vi "Scale Rotated Recangle.vi"(0 "Scaled(%)":sgl, 1 "Type":enum16{"Image", "Text"}(ring), 2 "Automatic":bool, 5 "Original Rectangle":cluster{"width":dbl, "height":dbl}, 7 "Angle (rad)":dbl, 9 "Page or text zone size":cluster{"width":dbl, "height":dbl}, 11 "error in (no error)":errorcluster) -> (4 "Scale Factor (%)":dbl, 6 "Scale Factor":dbl, 8 "Scaled Rectangle":cluster{"width":dbl, "height":dbl}, 10 "Offset":cluster{"X":dbl, "Y":dbl}, 15 "error out":errorcluster)   [LabVIEW 2013]
doc: "Version 1.0\nDeveloped by Jean-Marc Simard\nCopyright © 2010, Exaprom Inc.\nAll rights reserved.\nLicense: BSD"
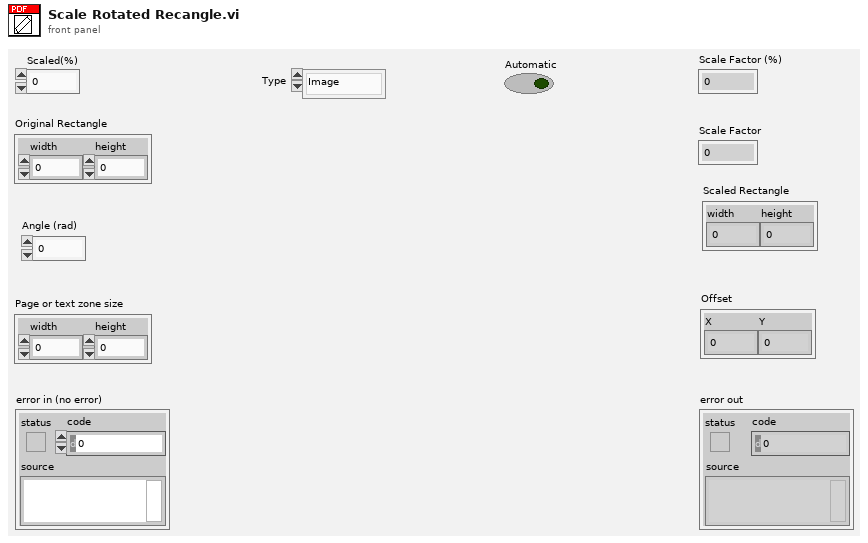
[diagram p1: front panel]
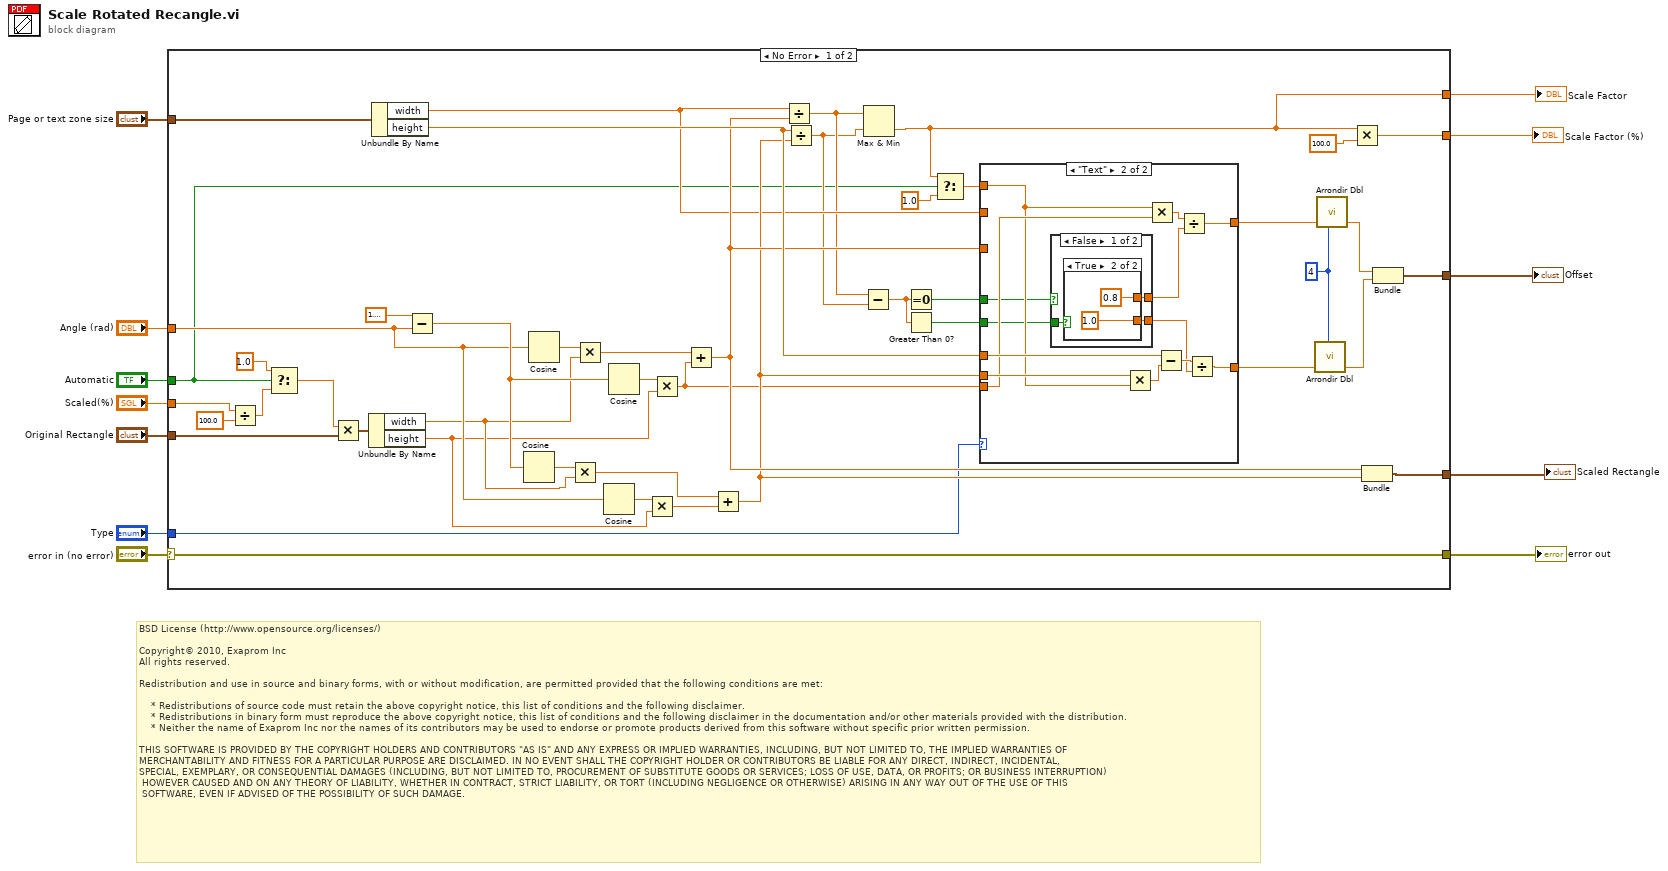
[diagram p0: block diagram]
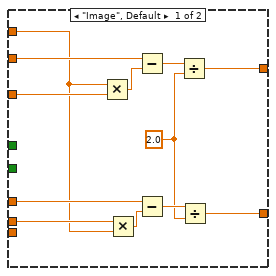
[diagram p2: hidden frame]
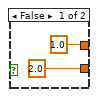
[diagram p3: hidden frame]
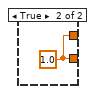
[diagram p4: hidden frame]
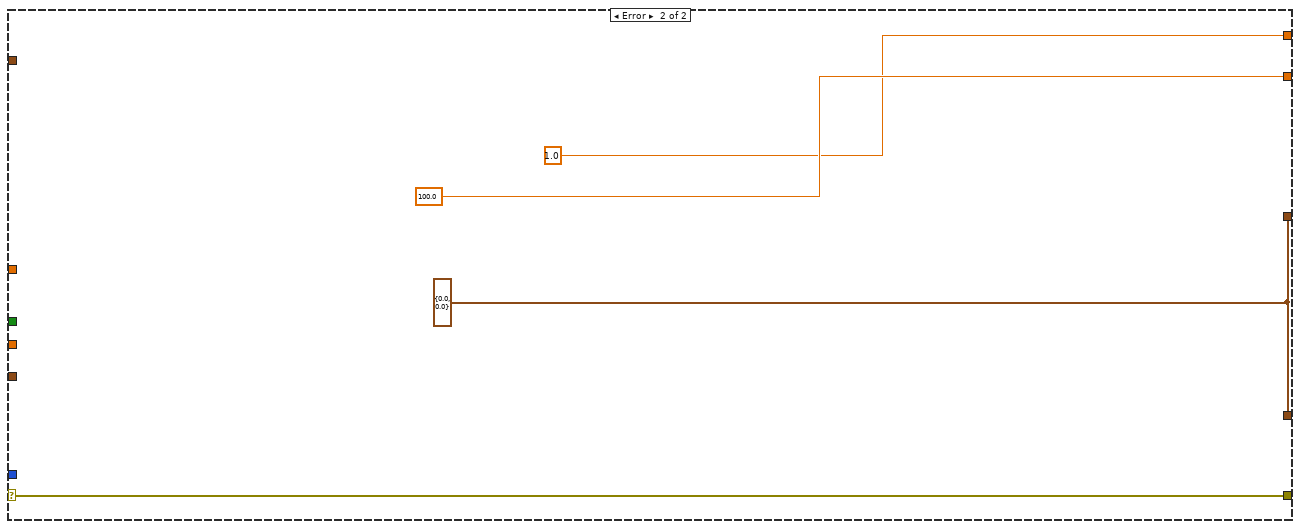
[diagram p5: hidden frame]
diagram:
  # "BSD License (http://www.opensource.org/licenses/)\n\nCopyright© 2010, Exaprom Inc\nAll rights reserved.\n\nRedistribution and use in source and binary forms, with or without modification, are permitted provided that the following conditions are met:\n\n    * Redistributions of source code must retain the above copyright notice, this list of conditions and the following disclaimer.\n    * Redistributions in binary form must reproduce the above copyright notice, this list of conditions and the following disclaimer in the documentation and/or other materials provided with the distribution.\n    * Neither the name of Exaprom Inc nor the names of its contributors may be used to endorse or promote products derived from this software without specific prior written permission.\n\nTHIS SOFTWARE IS PROVIDED BY THE COPYRIGHT HOLDERS AND CONTRIBUTORS \"AS IS\" AND ANY EXPRESS OR IMPLIED WARRANTIES, INCLUDING, BUT NOT LIMITED TO, THE IMPLIED WARRANTIES OF \nMERCHANTABILITY AND FITNESS FOR A PARTICULAR PURPOSE ARE DISCLAIMED. IN NO EVENT SHALL THE COPYRIGHT HOLDER OR CONTRIBUTORS BE LIABLE FOR ANY DIRECT, INDIRECT, INCIDENTAL,\nSPECIAL, EXEMPLARY, OR CONSEQUENTIAL DAMAGES (INCLUDING, BUT NOT LIMITED TO, PROCUREMENT OF SUBSTITUTE GOODS OR SERVICES; LOSS OF USE, DATA, OR PROFITS; OR BUSINESS INTERRUPTION)\n HOWEVER CAUSED AND ON ANY THEORY OF LIABILITY, WHETHER IN CONTRACT, STRICT LIABILITY, OR TORT (INCLUDING NEGLIGENCE OR OTHERWISE) ARISING IN ANY WAY OUT OF THE USE OF THIS\n SOFTWARE, EVEN IF ADVISED OF THE POSSIBILITY OF SUCH DAMAGE."
  n1 = case shown="No Error" "error in (no error)" {
    selector: "error in (no error)" -> [w57 w94]
    tunnel: [w57 w94] -> w12
    tunnel: "Original Rectangle" -> [w27 _]
    tunnel: "Angle (rad)" -> [w48 _]
    tunnel: [w47 w92] -> w8
    tunnel: "Page or text zone size" -> [w46 _]
    tunnel: [w32 100.0] -> w6
    tunnel: [w43 w92] -> w5
    tunnel: [w13 1.0] -> w4
    tunnel: "Type" -> [w31 _]
    tunnel: "Automatic" -> [w16 _]
    tunnel: "Scaled(%)" -> [w23 _]
    frame No Error {
      w34 = u8 4 ("Décimale")
      n2 = Divide(x=w23, y=sgl 100.0) -> (x/y=w25:sgl)
      n3 = Select(t=sgl 1.0 ("f"), s=w16, f=w25) -> (s? t:f=w22:sgl)
      n4 = Multiply(x=w22, y=w27) -> (x*y=w28:cluster{"width":dbl, "height":dbl})
      n5 = Unbundle By Name(w28) -> ("width"=w45:dbl, "height"=w41:dbl)
      n6 = Unbundle By Name(w46) -> ("width"=w39:dbl, "height"=w44:dbl)
      n7 = Subtract(x=1.5707963267948966, y=w48) -> (x-y=w49:dbl)
      n8 = Cosine(x=w49) -> (cos(x)=w50:dbl)
      n9 = Cosine(x=w48) -> (cos(x)=w55:dbl)
      n10 = Multiply(x=w50, y=w45) -> (x*y=w53:dbl)
      n11 = Multiply(x=w55, y=w45) -> (x*y=w30:dbl)
      n12 = Cosine(x=w48) -> (cos(x)=w51:dbl)
      n13 = Cosine(x=w49) -> (cos(x)=w54:dbl)
      n14 = Multiply(x=w51, y=w41) -> (x*y=w52:dbl)
      n15 = Multiply(x=w54, y=w41) -> (x*y=w29:dbl)
      n16 = Add(x=w30, y=w29) -> (x+y=w42:dbl)
      n17 = Add(x=w53, y=w52) -> (x+y=w40:dbl)
      n18 = Divide(x=w39, y=w42) -> (x/y=w21:dbl)
      n19 = Divide(x=w44, y=w40) -> (x/y=w20:dbl)
      n20 = Subtract(x=w21, y=w20) -> (x-y=w18:dbl)
      n21 = Max & Min(x=w21, y=w20) -> (min(x,y)=w13:dbl)  [unwired: 1 out]
      n22 = Equal To 0?(x=w18) -> (x = 0?=w19:bool)
      n23 = Greater Than 0?(x=w18) -> (x > 0?=w17:bool)
      n24 = Select(t=w13, s=w16, f=1.0 ("t")) -> (s? t:f=w15:dbl)
      n25 = case shown="\"Text\"" w31 {
        tunnel: w44 -> [w69 w82]
        tunnel: w42 -> [w65 _]
        tunnel: w40 -> [w64 w79]
        tunnel: w39 -> [w62 _]
        tunnel: [w60 w78] -> w38
        tunnel: [w59 w71] -> w37
        tunnel: w29 -> [_ w77]
        tunnel: w15 -> [w58 w76]
        tunnel: w19 -> [_ w75]
        tunnel: w17 -> [_ w74]
        frame "Image", Default {
          w66 = 2.0 ("y")
          n26 = Multiply(x=w58, y=w65) -> (x*y=w63:dbl)
          n27 = Multiply(x=w64, y=w58) -> (x*y=w68:dbl)
          n28 = Subtract(x=w62, y=w63) -> (x-y=w61:dbl)
          n29 = Subtract(x=w69, y=w68) -> (x-y=w67:dbl)
          n30 = Divide(x=w61, y=w66) -> (x/y=w59:dbl)
          n31 = Divide(x=w67, y=w66) -> (x/y=w60:dbl)
        }
        frame "Text" {
          n32 = case shown="False" w75 {
            tunnel: w74 -> [w85 _]
            tunnel: [w84 w90] -> w73
            tunnel: [w83 w90] -> w70
            frame False {
              n33 = case shown="True" w85 {
                tunnel: [2.0 ("y") 1.0 ("y")] -> w84
                tunnel: [1.0 ("y") 0.8 ("y")] -> w83
                frame False {
                }
                frame True {
                }
              }
            }
            frame True {
              w90 = 1.0 ("y")
            }
          }
          n34 = Multiply(x=w79, y=w76) -> (x*y=w81:dbl)
          n35 = Multiply(x=w76, y=w77) -> (x*y=w72:dbl)
          n36 = Subtract(x=w82, y=w81) -> (x-y=w80:dbl)
          n37 = Divide(x=w72, y=w70) -> (x/y=w71:dbl)
          n38 = Divide(x=w80, y=w73) -> (x/y=w78:dbl)
        }
      }
      n39 = call "Arrondir Dbl.vi"("Nombre IN"=w38, "Décimale"=w34) -> ("Nombre OUT"=w35:dbl)  [unwired: 5 out]
      n40 = call "Arrondir Dbl.vi"("Nombre IN"=w37, "Décimale"=w34) -> ("Nombre OUT"=w36:dbl)  [unwired: 5 out]
      n41 = Multiply(x=w13, y=100.0) -> (x*y=w32:dbl)
      n42 = Bundle(w42, w40) -> (w47:cluster{dbl, dbl})  [unwired: 1 out]
      n43 = Bundle("Nombre OUT"=w36, "Nombre OUT"=w35) -> (w43:cluster{"Nombre OUT":dbl, "Nombre OUT":dbl})  [unwired: 1 out]
    }
    frame Error {
      w92 = cluster{dbl, dbl} {0.0, 0.0}
    }
  }
  "error out" <- w12
  "Scaled Rectangle" <- w8
  "Scale Factor (%)" <- w6
  "Offset" <- w5
  "Scale Factor" <- w4
